vi "translate.vi"(0 "reference":refnum<class "RectangularNode.lvclass">, 1 "dx":dbl format="%.2f", 2 "dy":dbl format="%.2f", 5 "error in (no error)":errorcluster) -> (14 "reference out":refnum<class "RectangularNode.lvclass">, 19 "error out":errorcluster)   [LabVIEW 2014, in "RectangularNode.lvclass"]
doc: "public void translate(double dx, double dy)"
uses:
  <resource>/Framework/Providers/Open_GDS/UML/RectangularNode_class/RectangularNode.lvclass
  <resource>/Framework/Providers/Open_GDS/UML/AbstractNode_class/AbstractNode.lvclass
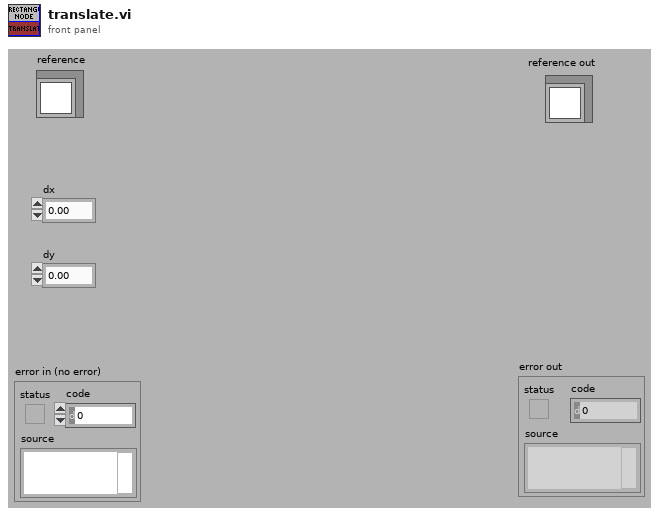
[diagram p1: front panel]
types:
  T1 = typedef "RectangularNode.lvclass/ObjectAttributes.ctl" = cluster{"bounds":T2}
  T2 = typedef "Rectangle Rectangle2D.ctl" = cluster{"x":dbl, "y":dbl, "width":dbl, "height":dbl}
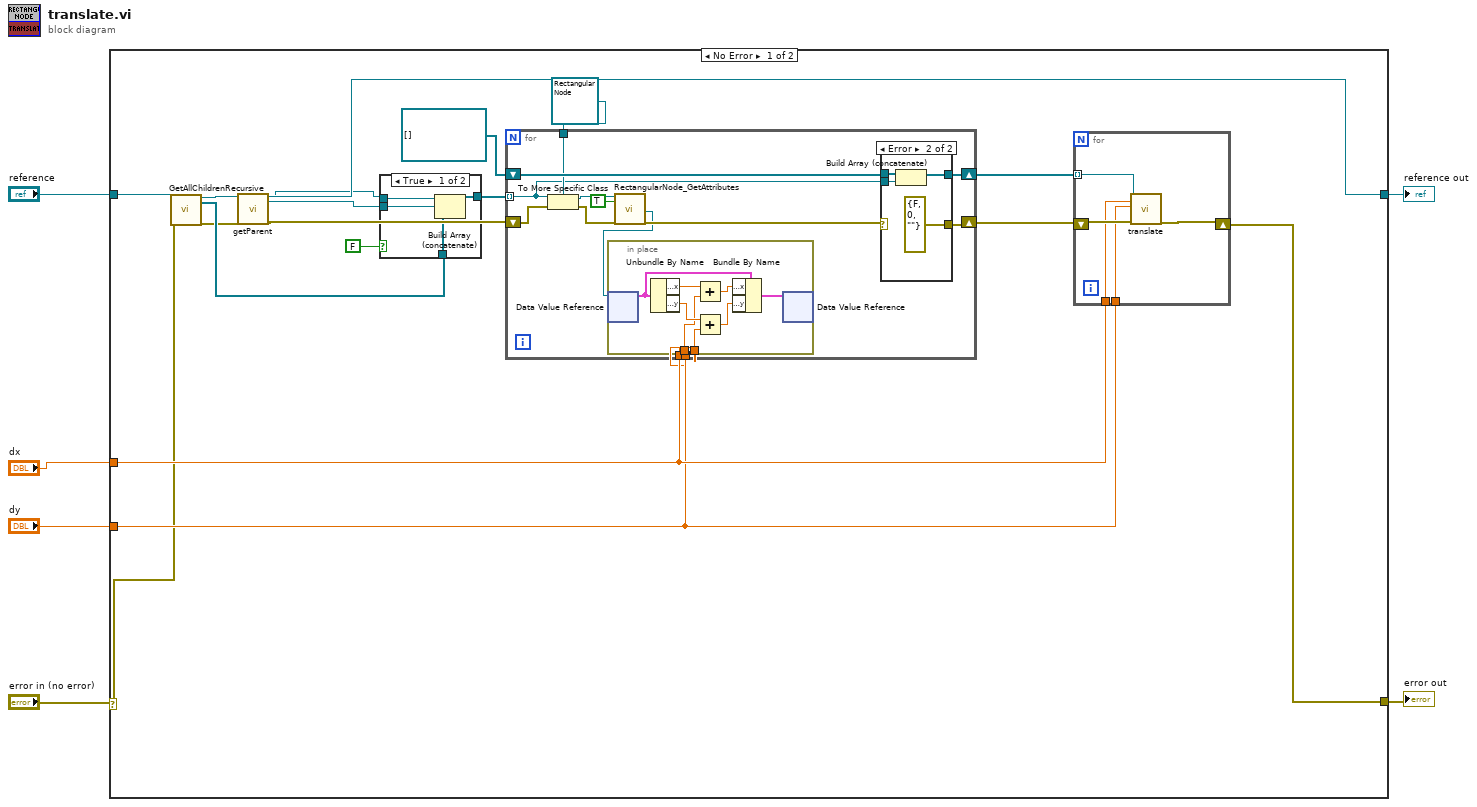
[diagram p0: block diagram]
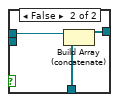
[diagram p2: hidden frame]
diagram:
  n1 = case shown="No Error" "error in (no error)" {
    selector: "error in (no error)" -> [w15 w63]
    tunnel: "reference" -> [w16 w64]
    tunnel: [w17 w63] -> w5
    tunnel: [w12 w64] -> w4
    tunnel: "dx" -> [w19 _]
    tunnel: "dy" -> [w18 _]
    frame No Error {
      n2 = call <resource>:"GetAllChildrenRecursive.vi"("reference"=w16, "error in (no error)"=w15) -> ("reference out"=w12:refnum<class "RectangularNode.lvclass">, "children"=w14:refnum<class "AbstractNode.lvclass">[], "error out"=w11:errorcluster)  [unwired: 15 out]
      n3 = call-dynamic "getParent.vi"("reference"=w12, "error in (no error)"=w11) -> ("reference out"=w9:refnum<class "RectangularNode.lvclass">, "parentNode"=w8:refnum<class "AbstractNode.lvclass">, "error out"=w10:errorcluster)  [unwired: 13 in, 2 out]
      n4 = case shown="True" FALSE {
        tunnel: [w32 w35] -> w23
        tunnel: w9 -> [w31 w34]
        tunnel: w14 -> [w30 w33]
        tunnel: w8 -> [w29 _]
        frame True {
          n5 = Build Array (concatenate)(w31, w29, w30) -> (w32:refnum<class "AbstractNode.lvclass">[])
        }
        frame False {
          n6 = Build Array (concatenate)(w34, w33) -> (w35:refnum<class "AbstractNode.lvclass">[])
        }
      }
      n7 = for {
        tunnel: w23 -> [w40] mode=indexing
        tunnel: w19 -> [w37]
        tunnel: w18 -> [w36]
        shift-right: [w47] -> w20
        shift-left: refnum<class "AbstractNode.lvclass">[] [] -> [w48]
        shift-right: [w45] -> w21
        shift-left: w10 -> [w42]
        tunnel: refnum<class "RectangularNode.lvclass"> refnum ("reference out") -> [w44]
        n8 = To More Specific Class(target class=w44, reference=w40, error in=w42) -> (specific class reference=w43:refnum<class "RectangularNode.lvclass">, error out=w41:errorcluster)
        n9 = call <resource>:"RectangularNode_GetAttributes.vi"("reference in"=w43, "OnlyGetDvrReference(False)"=TRUE, "error in (no error)"=w41) -> ("DataRef"=w38:refnum<data-value>, "error out"=w46:errorcluster)  [unwired: 13 in, 2 out]
        n10 = in-place {
          in-place-border: w37 -> [w50]
          in-place-border: w36 -> [w49]
          n11 = in-place-dvr #1(w38) -> (w56:T1)  [unwired: 1 out]
          n12 = Unbundle By Name(w56) -> ("bounds.x"=w55:dbl, "bounds.y"=w54:dbl)
          n13 = Add(x=w55, y=w50) -> (x+y=w53:dbl)
          n14 = Add(x=w54, y=w49) -> (x+y=w52:dbl)
          n15 = Bundle By Name(cluster=w56, "bounds.x"=w53, "bounds.y"=w52) -> (w51:T1)
          n16 = in-place-dvr #1(w51) -> ()  [unwired: 2 out]
        }
        n17 = case shown="Error" w46 {
          selector: w46 -> [w58 _]
          tunnel: w48 -> [w57 w62]
          tunnel: [w57 w61] -> w47
          tunnel: [w58 errorcluster {"status"=FALSE, "code"=0, "source"=""} ("error IO")] -> w45
          tunnel: w40 -> [_ w59]
          frame No Error {
          }
          frame Error {
            n18 = Build Array (concatenate)(w62, w59) -> (w61:refnum<class "AbstractNode.lvclass">[])
          }
        }
      }
      n19 = for {
        shift-right: [w27] -> w17
        shift-left: w21 -> [w28]
        tunnel: w20 -> [w26] mode=indexing
        tunnel: w19 -> [w25]
        tunnel: w18 -> [w24]
        n20 = call-dynamic "translate.vi"("reference"=w26, "dx"=w25, "dy"=w24, "error in (no error)"=w28) -> ("error out"=w27:errorcluster)  [unwired: 14 in, 1 out]
      }
    }
    frame Error {
    }
  }
  "reference out" <- w4
  "error out" <- w5
